vi "Format StartInstancesResult_LVXML_InstancesSet.vi"(8 "error in (no error)":errorcluster, 11 "Siblings":T4(array[cluster])) -> (0 "error out":errorcluster, 3 "Array":T1[](array[typedef]))   [LabVIEW 2014, in "AWS_EC2.lvlib" / "AWS_EC2.lvclass"]
uses:
  AWS_EC2.lvclass
  lv-xml-parser/r0/trunk/VI Source/EventType.ctl
  EC2 Datatypes/InstanceStateChangeSetType.ctl
  EC2 Datatypes/InstanceStateType.ctl
  AWS_EC2.lvlib
  lv-xml-parser/r0/trunk/VI Source/LV XML Parser.lvlib
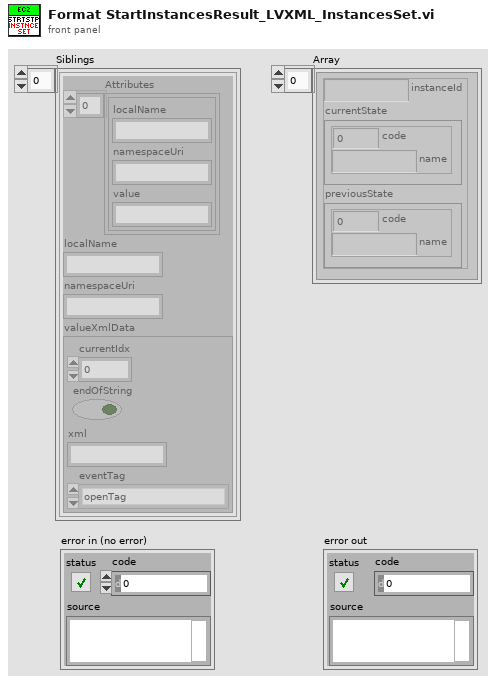
[diagram p1: front panel]
types:
  T1 = typedef "AWS_EC2.lvlib/InstanceStateChangeSetType.ctl" = cluster{"instanceId":string, "currentState":T2, "previousState":T2}
  T2 = typedef "AWS_EC2.lvlib/InstanceStateType.ctl" = cluster{"code":i16, "name":string}
  T3 = typedef "LV XML Parser.lvlib/EventType.ctl" = enum16{"openTag", "endOpenTag", "closeTag", "comment", "endComment", "endOfFile", "attribute", "startXml"}
  T4 = cluster{"Attributes":cluster{"localName":string, "namespaceUri":string, "value":string}[], "localName":string, "namespaceUri":string, "valueXmlData":cluster{"currentIdx":i32, "endOfString":bool, "xml":string, "eventTag":T3}}[]
  T5 = cluster{"Attributes":cluster{"localName":string, "namespaceUri":string, "value":string}[], "localName":string, "namespaceUri":string, "valueXmlData":cluster{"currentIdx":i32, "endOfString":bool, "xml":string, "eventTag":T3}}
  T6 = cluster{"currentIdx":i32, "endOfString":bool, "xml":string, "eventTag":T3}
  T7 = cluster{"namespaceUri":string, "localName":string}
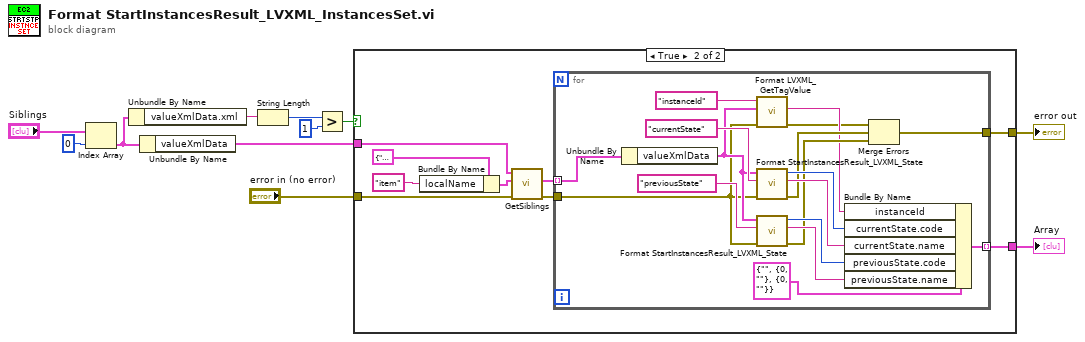
[diagram p0: block diagram]
diagram:
  n1 = Index Array(array="Siblings", index=0) -> (element=w1:T5)
  n2 = Unbundle By Name(w1) -> ("valueXmlData.xml"=w2:string)
  n3 = Unbundle By Name(w1) -> ("valueXmlData"=w3:T6)
  n4 = String Length(string=w2) -> (length=w6:i32)
  n5 = Greater?(x=w6, y=1) -> (0:w4:bool)
  n6 = case shown="True" w4 {
    tunnel: [w12 w20] -> w11
    tunnel: [_ w19] -> w10
    tunnel: "error in (no error)" -> [w12 w14]
    tunnel: w3 -> [_ w13]
    frame False {
    }
    frame True {
      n7 = Bundle By Name(cluster=T7 {"namespaceUri"="", "localName"=""} ("limitToTag"), "localName"="item" ("Tag name")) -> (w16:T7)
      n8 = call "GetSiblings.vi"("error in (no error)"=w14, "limitToTag"=w16, "xmlData"=w13) -> ("error out"=w21:errorcluster, "Siblings"=w17:T4)  [unwired: 7 in]
      n9 = for {
        tunnel: w17 -> [w33] mode=indexing
        tunnel: [w35] -> w19 mode=indexing
        tunnel: [w27] -> w20
        tunnel: w21 -> [w24]
        n10 = Unbundle By Name(w33) -> ("valueXmlData"=w25:T6)
        n11 = call "Format LVXML_GetTagValue.vi"("error in (no error)"=w24, "xmlDataIn"=w25, "Tag name"="instanceId") -> ("error out"=w22:errorcluster, "Value"=w23:string)  [unwired: 6 in, 1 out]
        n12 = call "Format StartInstancesResult_LVXML_State.vi"("error in (no error)"=w24, "State Tag"="currentState" ("Tag name"), "valueXmlData"=w25) -> ("error out"=w29:errorcluster, "State.name"=w34:string, "State.code"=w36:i16)  [unwired: 6 in]
        n13 = call "Format StartInstancesResult_LVXML_State.vi"("error in (no error)"=w24, "State Tag"="previousState" ("Tag name"), "valueXmlData"=w25) -> ("error out"=w28:errorcluster, "State.name"=w30:string, "State.code"=w31:i16)  [unwired: 6 in]
        n14 = Bundle By Name(cluster=T1 {"instanceId"="", "currentState"={"code"=0, "name"=""}, "previousState"={"code"=0, "name"=""}} ("InstanceStateChangeSetType"), "instanceId"=w23, "currentState.code"=w36, "currentState.name"=w34, "previousState.code"=w31, "previousState.name"=w30) -> (w35:T1)
        n15 = Merge Errors(w22, w29, w28) -> (w27:errorcluster)
      }
    }
  }
  "error out" <- w11
  "Array" <- w10
